vi "SortFilesByDate.vi"(1 "directory path":path) -> (0 "Files by date":cluster{"Time Stamp":u32, "File Name":string}[](array[cluster]) {"Time Stamp" format="%<%I:%M:%S %p\n%m/%d/%Y>T"})   [LabVIEW 2012]
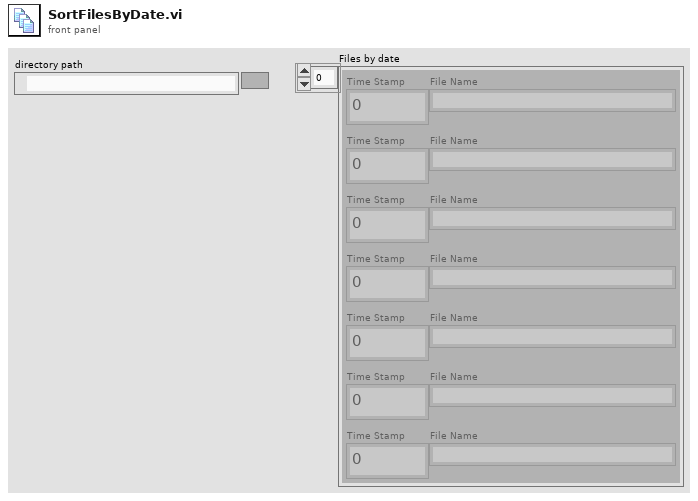
[diagram p1: front panel]
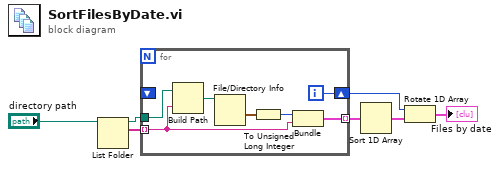
[diagram p0: block diagram]
diagram:
  n1 = List Folder(path="directory path") -> (path out=w6:path, filenames=w7:string[])  [unwired: 3 in, 2 out]
  n2 = for {
    tunnel: w7 -> [w10] mode=indexing
    tunnel: w6 -> [w14]
    tunnel: [w12] -> w5 mode=indexing
    shift-right: [w8] -> w1
    shift-left: _ -> [_]
    i -> [w8]
    n3 = Build Path(base path=w14, name or relative path=w10) -> (appended path=w11:path)
    n4 = File/Directory Info(path=w11) -> (last mod=w9:timestamp)  [unwired: 1 in, 6 out]
    n5 = To Unsigned Long Integer(number=w9) -> (unsigned 32bit integer=w13:u32)
    n6 = Bundle(w13, w10) -> (w12:cluster{u32, string})  [unwired: 1 in]
  }
  n7 = Sort 1D Array(array=w5) -> (sorted array=w2:cluster{u32, string}[])
  n8 = Rotate 1D Array(1:w2, 2:w1) -> (0:→"Files by date":cluster{u32, string}[])
